vi "_Set DC Line.vi"(2 "States":u8, 3 "DC Line":T1) -> ()   [LabVIEW 2012]
uses:
  Type/_FPGA DC Lines.ctl
  Type/_FPGA Chip Type.ctl
  <vilib>/rvi/eio/common/nirviEmuTemplateMethod_errors.vi
  <vilib>/eio/EIONode/EIONode.xnode
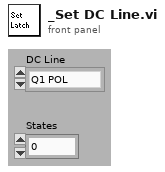
[diagram p1: front panel]
types:
  T1 = typedef "_FPGA DC Lines.ctl" = enum16{"Q1 POL", "Q3 POL", "Q1 DC EN", "Q3 DC EN", "COR POL", "CUR POL", "S1 POL", "S2 POL", "CEM POL"}
  T2 = typedef "_FPGA Chip Type.ctl" = enum8{"None", "ADC1", "ADC2", "ADC3", "ADC4", "ADC5", "ADC6", "ADC7", "ADC8", "ADC9", "ADC10", "ADC11", "ADC12", "ADC13", "DAC1", "DAC2", "DAC3", "DAC4", "DAC5", "LENS1", "LENS2", "LENS3", "LENS4", "LENS5", "LENS6", "LENS7", "MASS1", "MASS2", "MASS3", "MASS4", "MASS5", "OSC1", "OSC2", "OSC3", "LATCH1", "LATCH2", "LATCH3", "LATCH4", "PIC1", "PIC2", "PIC3", "PIC4"}
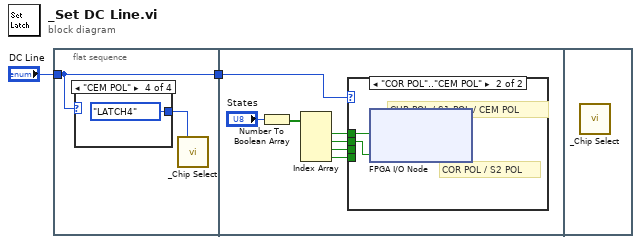
[diagram p0: block diagram]
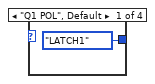
[diagram p2: hidden frame]
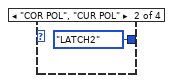
[diagram p3: hidden frame]
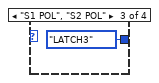
[diagram p4: hidden frame]
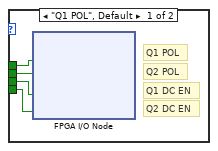
[diagram p5: hidden frame]
diagram:
  n1 = flat-sequence {
    tunnel: [w3] -> w2
    tunnel: "DC Line" -> [w3]
    tunnel: w2 -> [w15]
    frame #0 {
      n2 = case shown="\"CEM POL\"" w3 {
        tunnel: [_FPGA_Chip_Type."LATCH1" ("ChipType") _FPGA_Chip_Type."LATCH2" ("ChipType") _FPGA_Chip_Type."LATCH3" ("ChipType") _FPGA_Chip_Type."LATCH4" ("ChipType")] -> w4
        frame "Q1 POL", Default {
        }
        frame "COR POL", "CUR POL" {
        }
        frame "S1 POL", "S2 POL" {
        }
        frame "CEM POL" {
        }
      }
      n3 = call "_Chip Select.vi"("ChipType"=w4) -> ()  [unwired: 1 in, 6 out]
    }
    frame #1 {
      n4 = Number To Boolean Array(number="States") -> (Boolean array=w13:bool[])
      n5 = Index Array(array=w13) -> (element #1=w12:bool, element #2=w11:bool, element #3=w10:bool, element #4=w9:bool)  [unwired: 4 in]
      n6 = case shown="\"COR POL\"..\"CEM POL\"" w15 {
        tunnel: w12 -> [w16 w21]
        tunnel: w11 -> [w19 w20]
        tunnel: w10 -> [w18 _]
        tunnel: w9 -> [w17 _]
        frame "Q1 POL", Default {
          # "Q2 DC EN"
          # "Q1 DC EN"
          # "Q2 POL"
          # "Q1 POL"
          n7 = xnode "FPGA I/O Node"("Port4/DIO6"=w16, "Port4/DIO5"=w19, "Port4/DIO4"=w18, "Port4/DIO3"=w17) -> ()  [unwired: 4 in, 4 out]
        }
        frame "COR POL".."CEM POL" {
          # "COR POL / S2 POL"
          # "CUR POL / S1 POL / CEM POL"
          n8 = xnode "FPGA I/O Node"("Port4/DIO0"=w21, "Port3/DIO8"=w20) -> ()  [unwired: 2 in, 2 out]
        }
      }
    }
    frame #2 {
      n9 = call "_Chip Select.vi"() -> ()  [unwired: 2 in, 6 out]
    }
  }
